vi "ShutterClose.vi"(8 "error in (no error)":errorcluster, 10 "Shutter number":i32, 11 "Microscope in":refnum<class "Microscope.lvclass">) -> (0 "error out":errorcluster, 3 "Microscope out":refnum<class "Microscope.lvclass">)   [LabVIEW 2012, in "Microscope.lvclass"]
uses:
  classes/Microscope.lvclass
  classes/Microscope.lvclass/Microscope.ctl
  <vilib>/DAQmx/write.llb/DAQmx Write (Digital Bool 1Line 1Point).vi
  <vilib>/DAQmx/create/channels.llb/DAQmx Create Channel (DO-Digital Output).vi
  <vilib>/DAQmx/miscellaneous.llb/DAQmx Fill In Error Info.vi
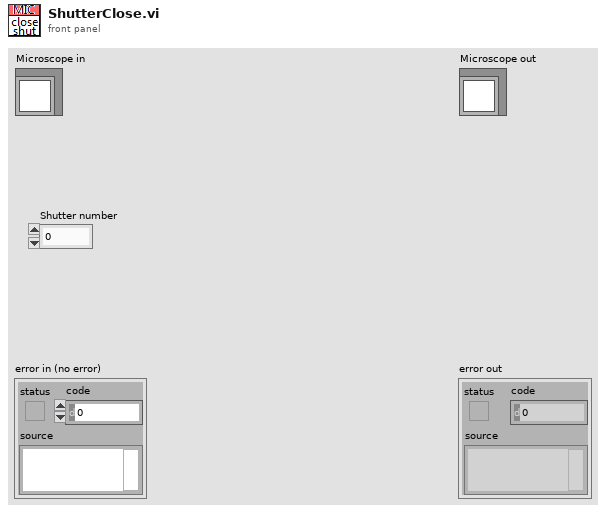
[diagram p1: front panel]
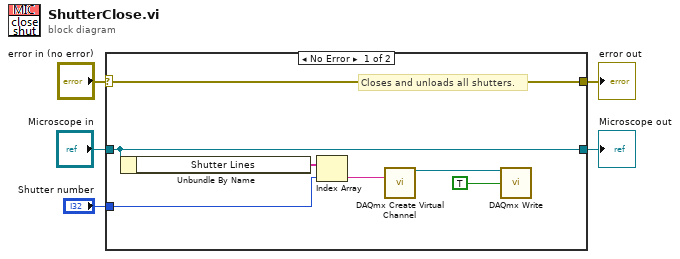
[diagram p0: block diagram]
diagram:
  n1 = case shown="No Error" "error in (no error)" {
    selector: "error in (no error)" -> [w12 w14]
    tunnel: [w12 w14] -> w4
    tunnel: [w8 w13] -> w2
    tunnel: "Microscope in" -> [w8 w13]
    tunnel: "Shutter number" -> [w9 _]
    frame No Error {
      # "Closes and unloads all shutters."
      n2 = Unbundle By Name(w8) -> ("Shutter Lines"=w10:tag[])
      n3 = Index Array(array=w10, index=w9) -> (element=w6:tag)
      n4 = call-poly <vilib>:"DAQmx Create Virtual Channel.vi"("lines"=w6) -> ("task out"=w7:refnum<k21>)  [unwired: 13 in, 1 out]
      n5 = call-poly <vilib>:"DAQmx Write.vi"("task/channels in"=w7, "data"=TRUE) -> ()  [unwired: 11 in, 3 out]
    }
    frame Error {
    }
  }
  "error out" <- w4
  "Microscope out" <- w2
